vi "ScanString.vi"(8 "error in (no error)":errorcluster, 10 "String":string, 11 "String dropdown D Element in":refnum<class "String dropdown D Element.lvclass">) -> (0 "error out":errorcluster, 3 "String dropdown D Element out":refnum<class "String dropdown D Element.lvclass">)   [LabVIEW 2020, in "D Datagrid Library.lvlib" / "String dropdown D Element.lvclass"]
uses:
  String dropdown D Element.lvclass
  String dropdown D Element.lvclass/String dropdown D Element.ctl
  4b7b142e-2c3c-4033-9d0a-c019c938586b.vi
  <vilib>/Comparison/Equal/Equal Functor/Equal Functor.lvclass
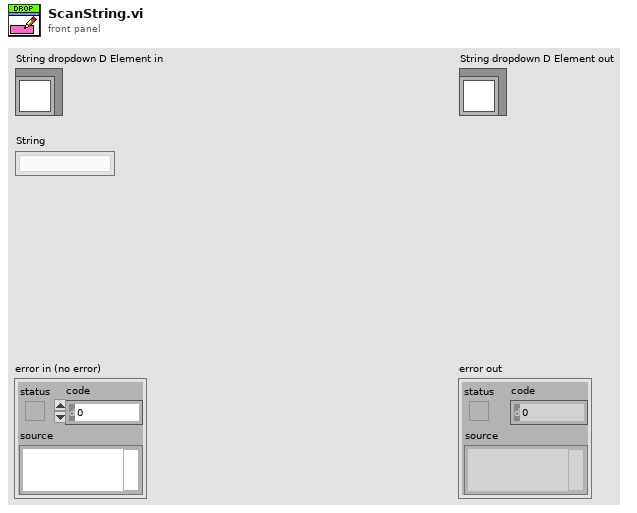
[diagram p1: front panel]
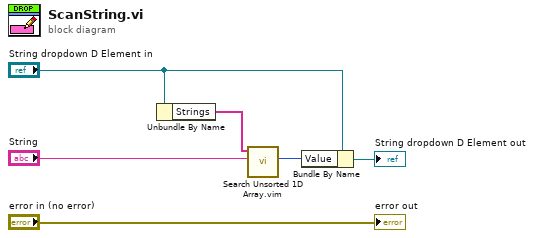
[diagram p0: block diagram]
diagram:
  n1 = Unbundle By Name("String dropdown D Element in") -> ("Strings"=w6:string[])
  n2 = call "Search Unsorted 1D Array.vim"("element"="String", "unsorted 1D array"=w6) -> ("index of element"=w2:i32)  [unwired: 9 in]
  n3 = Bundle By Name(cluster="String dropdown D Element in", "Value"=w2) -> (→"String dropdown D Element out":refnum<class "String dropdown D Element.lvclass">)
  "error out" <- "error in (no error)"
